vi "MM6Archiver.new data description.vi"(0 "i ref":refnum<vi>, 1 "dataDescription":string, 2 "descriptor":string, 3 "ms timeout (10000)":i32=10000, 5 "error in (no error)":errorcluster) -> (14 "i ref out":refnum<vi>, 17 "timed out":bool, 19 "error out":errorcluster)   [LabVIEW 2014, in "MM6Archiver.lvlib"]
doc: "The method is executed, when a dataDescription for a new run is received. In case the \"dataDescription\" is really new, the DiscArchiver will switch to a new file."
uses:
  MM6Archiver.lvlib
  CSCore/CSSystem/CoreDefs/CoreDefs.rawDataType.ctl
  CSData/DiscArchiver/DiscArchiver.lvlib
  CSData/DataLib/DataLib.lvlib
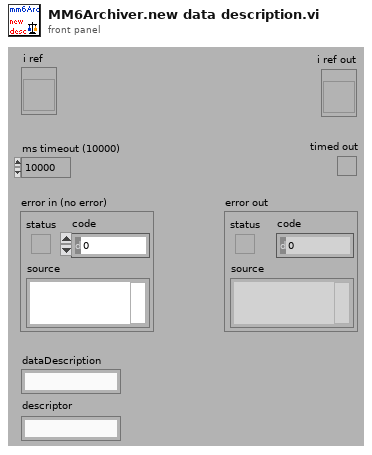
[diagram p1: front panel]
types:
  T1 = typedef "CoreDefs.rawDataType.ctl" = i8[]
  T2 = typedef "DiscArchiver.lvlib/DiscArchiver.i attribute.ctl" = cluster{"file prefix":string, "actual file":string, "nOfEvents":i32, "file":refnum<file>, "eventBuilder":string, "disc size alarm":bool, "dataDescription":string, "dataDescriptionURL":string, "eventDataURL":string, "headerID":dbl, "completeData":bool, "nOfEventsID":i32, "dataFileID":i32}
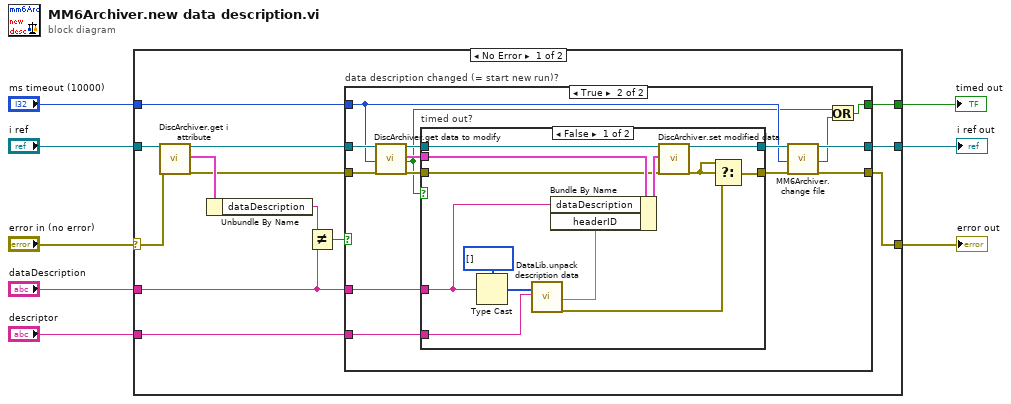
[diagram p0: block diagram]
diagram:
  n1 = case shown="No Error" "error in (no error)" {
    selector: "error in (no error)" -> [w18 w54]
    tunnel: [w11 w54] -> w8
    tunnel: "dataDescription" -> [w13 _]
    tunnel: [w10 w55] -> w6
    tunnel: "i ref" -> [w19 w55]
    tunnel: "ms timeout (10000)" -> [w14 _]
    tunnel: "descriptor" -> [w12 _]
    tunnel: [w9 _] -> w1
    frame No Error {
      n2 = call "DiscArchiver.get i attribute.vi"("i ref in"=w19, "error in (no error)"=w18) -> ("i ref out"=w16:refnum<vi>, "i attribute"=w20:T2, "error out"=w15:errorcluster)  [unwired: 15 in]
      n3 = Unbundle By Name(w20) -> ("dataDescription"=w21:string)
      n4 = Not Equal?(x=w21, y=w13) -> (x != y?=w17:bool)
      n5 = case "data description changed (= start new run)?" shown="True" w17 {
        tunnel: w16 -> [w23 w38]
        tunnel: w15 -> [w22 w37]
        tunnel: w14 -> [_ w29]
        tunnel: w13 -> [_ w34]
        tunnel: w12 -> [_ w33]
        tunnel: [w22 w28] -> w11
        tunnel: [w23 w27] -> w10
        tunnel: [_ w26] -> w9
        frame False {
        }
        frame True {
          n6 = call "DiscArchiver.get data to modify.vi"("i ref in"=w38, "ms timeout (10000)"=w29, "error in (no error)"=w37) -> ("i ref out"=w36:refnum<vi>, "i attribute"=w35:T2, "timed out"=w25:bool, "error out"=w32:errorcluster)  [unwired: 13 in]
          n7 = case "timed out?" shown="False" w25 {
            tunnel: w36 -> [w51 w52]
            tunnel: w35 -> [w50 _]
            tunnel: w34 -> [w48 _]
            tunnel: w33 -> [w49 _]
            tunnel: w32 -> [w43 w53]
            tunnel: [w42 w53] -> w30
            tunnel: [w39 w52] -> w31
            frame False {
              n8 = Type Cast(type=T1 [] ("Array"), x=w48) -> (*(type *) &x=w46:T1)
              n9 = call "DataLib.unpack description data.vi"("serviceData"=w46, "descriptor"=w49) -> ("headerID"=w45:dbl, "error out"=w40:errorcluster)  [unwired: 14 in, 2 out]
              n10 = Bundle By Name(cluster=w50, "dataDescription"=w48, "headerID"=w45) -> (w44:T2)
              n11 = call "DiscArchiver.set modified data.vi"("i ref in"=w51, "i attribute"=w44, "error in (no error)"=w43) -> ("i ref out"=w39:refnum<vi>, "error out"=w41:errorcluster)  [unwired: 15 in]
              n12 = Select(t=w41, s=w41, f=w40) -> (s? t:f=w42:errorcluster)
            }
            frame True {
            }
          }
          n13 = call "MM6Archiver.change file.vi"("i ref in"=w31, "ms timeout (10000)"=w29, "error in (no error)"=w30) -> ("i ref out"=w27:refnum<vi>, "timed out"=w24:bool, "error out"=w28:errorcluster)  [unwired: 14 in]
          n14 = Or(x=w25, y=w24) -> (x .or. y?=w26:bool)
        }
      }
    }
    frame Error {
    }
  }
  "error out" <- w8
  "i ref out" <- w6
  "timed out" <- w1
